vi "execute.vi"(8 "error in (no error)":errorcluster, 10 "Context in":refnum<class "Context.lvclass">, 11 "Command in":refnum<class "Command.lvclass">) -> (0 "error out":errorcluster, 2 "Context out":refnum<class "Context.lvclass">, 3 "Command out":refnum<class "Command.lvclass">)   [LabVIEW 2016, in "Command.lvclass"]
uses:
  Command.lvclass
  Context/Context/Context.lvclass
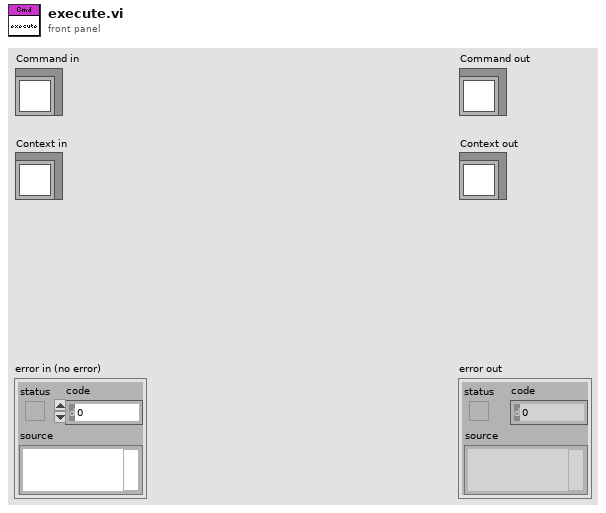
[diagram p1: front panel]
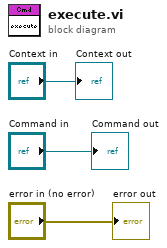
[diagram p0: block diagram]
diagram:
  "error out" <- "error in (no error)"
  "Command out" <- "Command in"
  "Context out" <- "Context in"
